vi "PD SYNC.vi"() -> ()   [LabVIEW 2017]
uses:
  <userlib>/Keithley 2000 Series (3.0.0) LV8.0+/Public/Configure/Configure DC Volts.vi
  <userlib>/Keithley 2000 Series (3.0.0) LV8.0+/Keithley 2000.lvlib
panel:
  in  "stop":bool
  out "Measurement":dbl
  out "Units":string
  in  "Custom Count (1)":i32=1
  in  "Power Line Cycles (1.00)":dbl=1.0 format="%.2f"
  in  "VISA resource name":refnum<visa-resource-name>="GPIB::16"
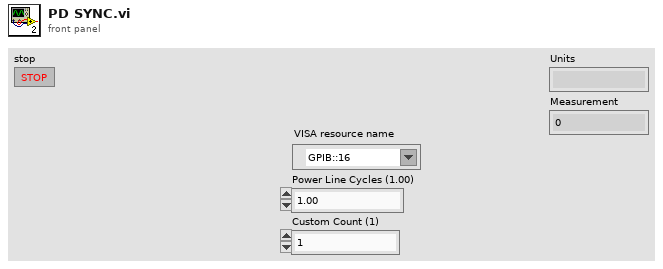
[diagram p1: front panel]
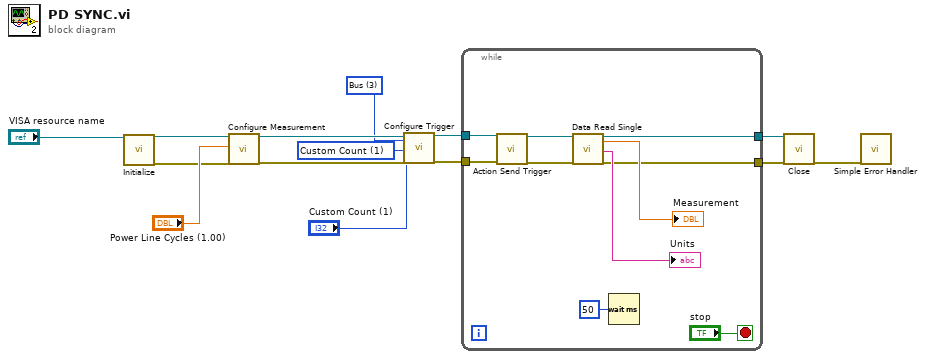
[diagram p0: block diagram]
diagram:
  w7 = u16 1 items=["Infinite", "Custom Count"] ("Count Mode (0: Infinite)")
  w8 = u16 3 items=["Immediate", "Timer", "Manual", "Bus", "External"] ("Source (0: Immediate)")
  n1 = call <userlib>:"Initialize.vi"("VISA resource name"="VISA resource name") -> ("VISA resource name out"=w13:refnum<visa-resource-name>, "error out"=w10:errorcluster)  [unwired: 17 in]
  n2 = call-poly <userlib>:"Configure Measurement.vi"("VISA resource name"=w13, "Power Line Cycles (1.00)"="Power Line Cycles (1.00)", "error in (no error)"=w10) -> ("VISA resource name out"=w11:refnum<visa-resource-name>, "error out"=w9:errorcluster)  [unwired: 15 in]
  n3 = call <userlib>:"Configure Trigger.vi"("VISA resource name"=w11, "Source (0: Immediate)"=w8, "Count Mode (0: Infinite)"=w7, "Custom Count (1)"="Custom Count (1)", "error in (no error)"=w9) -> ("VISA resource name out"=w5:refnum<visa-resource-name>, "error out"=w4:errorcluster)  [unwired: 13 in]
  n4 = while {
    tunnel: w5 -> [w24]
    tunnel: w4 -> [w23]
    tunnel: [w18] -> w3
    tunnel: [w17] -> w2
    stop <- "stop" stop-if-true
    n5 = call <userlib>:"Action Send Trigger.vi"("VISA resource name"=w24, "error in (no error)"=w23) -> ("VISA resource name out"=w22:refnum<visa-resource-name>, "error out"=w21:errorcluster)  [unwired: 16 in]
    n6 = call <userlib>:"Data Read Single.vi"("VISA resource name"=w22, "error in (no error)"=w21) -> ("VISA resource name out"=w18:refnum<visa-resource-name>, "Measurement"=→"Measurement":dbl, "Units"=→"Units":string, "error out"=w17:errorcluster)  [unwired: 13 in, 1 out]
    n7 = Wait (ms)(milliseconds to wait=u32 50) -> ()  [unwired: 1 out]
  }
  n8 = call <userlib>:"Close.vi"("VISA resource name"=w3, "error in (no error)"=w2) -> ("error out"=w1:errorcluster)  [unwired: 17 in]
  n9 = call <vilib>:"Simple Error Handler.vi"("error in (no error)"=w1) -> ()  [unwired: 4 in, 5 out]
